vi "Controller Test Bench (4).vi"() -> ()   [LabVIEW 2022 SP3]
uses:
  <vilib>/sound2/lvsound2.llb/Sound Data Format.ctl
  <vilib>/Utility/error.llb/DialogType.ctl
  <vilib>/sound2/lvsound2.llb/Sampling Mode.ctl
  <vilib>/Analysis/4window.llb/windowTd.ctl
  <vilib>/DAQmx/read.llb/DAQmx Read (Analog 1D Wfm NChan NSamp).vi
  <vilib>/DAQmx/write.llb/DAQmx Write (Analog 1D DBL 1Chan NSamp).vi
  <vilib>/DAQmx/create/channels.llb/DAQmx Create Channel (AO-Voltage-Basic).vi
  <vilib>/DAQmx/create/channels.llb/DAQmx Create Channel (AI-Acceleration-Accelerometer).vi
  <vilib>/DAQmx/configure/timing.llb/DAQmx Timing (Sample Clock).vi
  <vilib>/DAQmx/miscellaneous.llb/DAQmx Fill In Error Info.vi
  <vilib>/DAQmx/configure/task.llb/DAQmx Configure Logging (TDMS).vi
  <vilib>/measure/maspectr.llb/FFT Spectrum (Mag-Phase) for N Chan.vi
  <vilib>/sound2/lvsound2.llb/Sound Output Set Volume (Single).vi
  <vilib>/sound2/lvsound2.llb/Sound Output Write (DBL Single).vi
  <vilib>/measure/NI_MAPro.lvlib
  <resource>/objmgr/daqmx.rc
  <vilib>/Analysis/NI_AALPro.lvlib
panel:
  out "number of samples written per channel":u32
  in  "Active Control":bool
  in  "Output Noise":bool
  in  "Log Data":bool
  out "Phase 2":cluster{"f0":dbl, "df":dbl, "phase":dbl[]}[](graph)
  out "Mag 2":cluster{"f0":dbl, "df":dbl, "magnitude":dbl[]}[](graph)
  in  "Show FFT":bool
  in  "Save FFT":bool
  in  "Start Acquisition":bool
  in  "Stop":bool
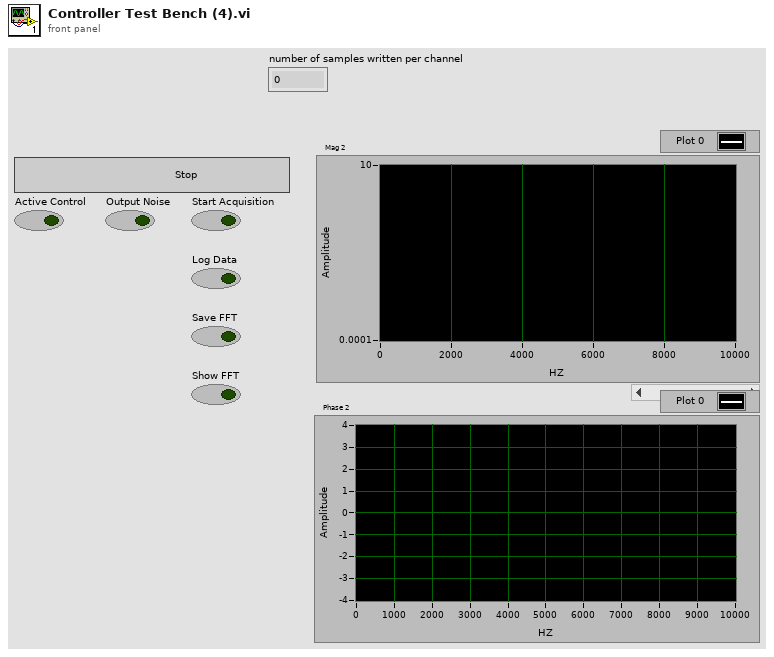
[diagram p1: front panel]
types:
  T1 = typedef "Sampling Mode.ctl" = i32
  T2 = typedef "DialogType.ctl" = u16
  T3 = typedef "Sound Data Format.ctl" = cluster{"sample rate (S/s)":dbl, "number of channels":i32, "bits per sample":i32}
  T4 = typedef "Sound Output Task ID.ctl" = u32
  T5 = typedef "NI_AALPro.lvlib/windowTd.ctl" = u32
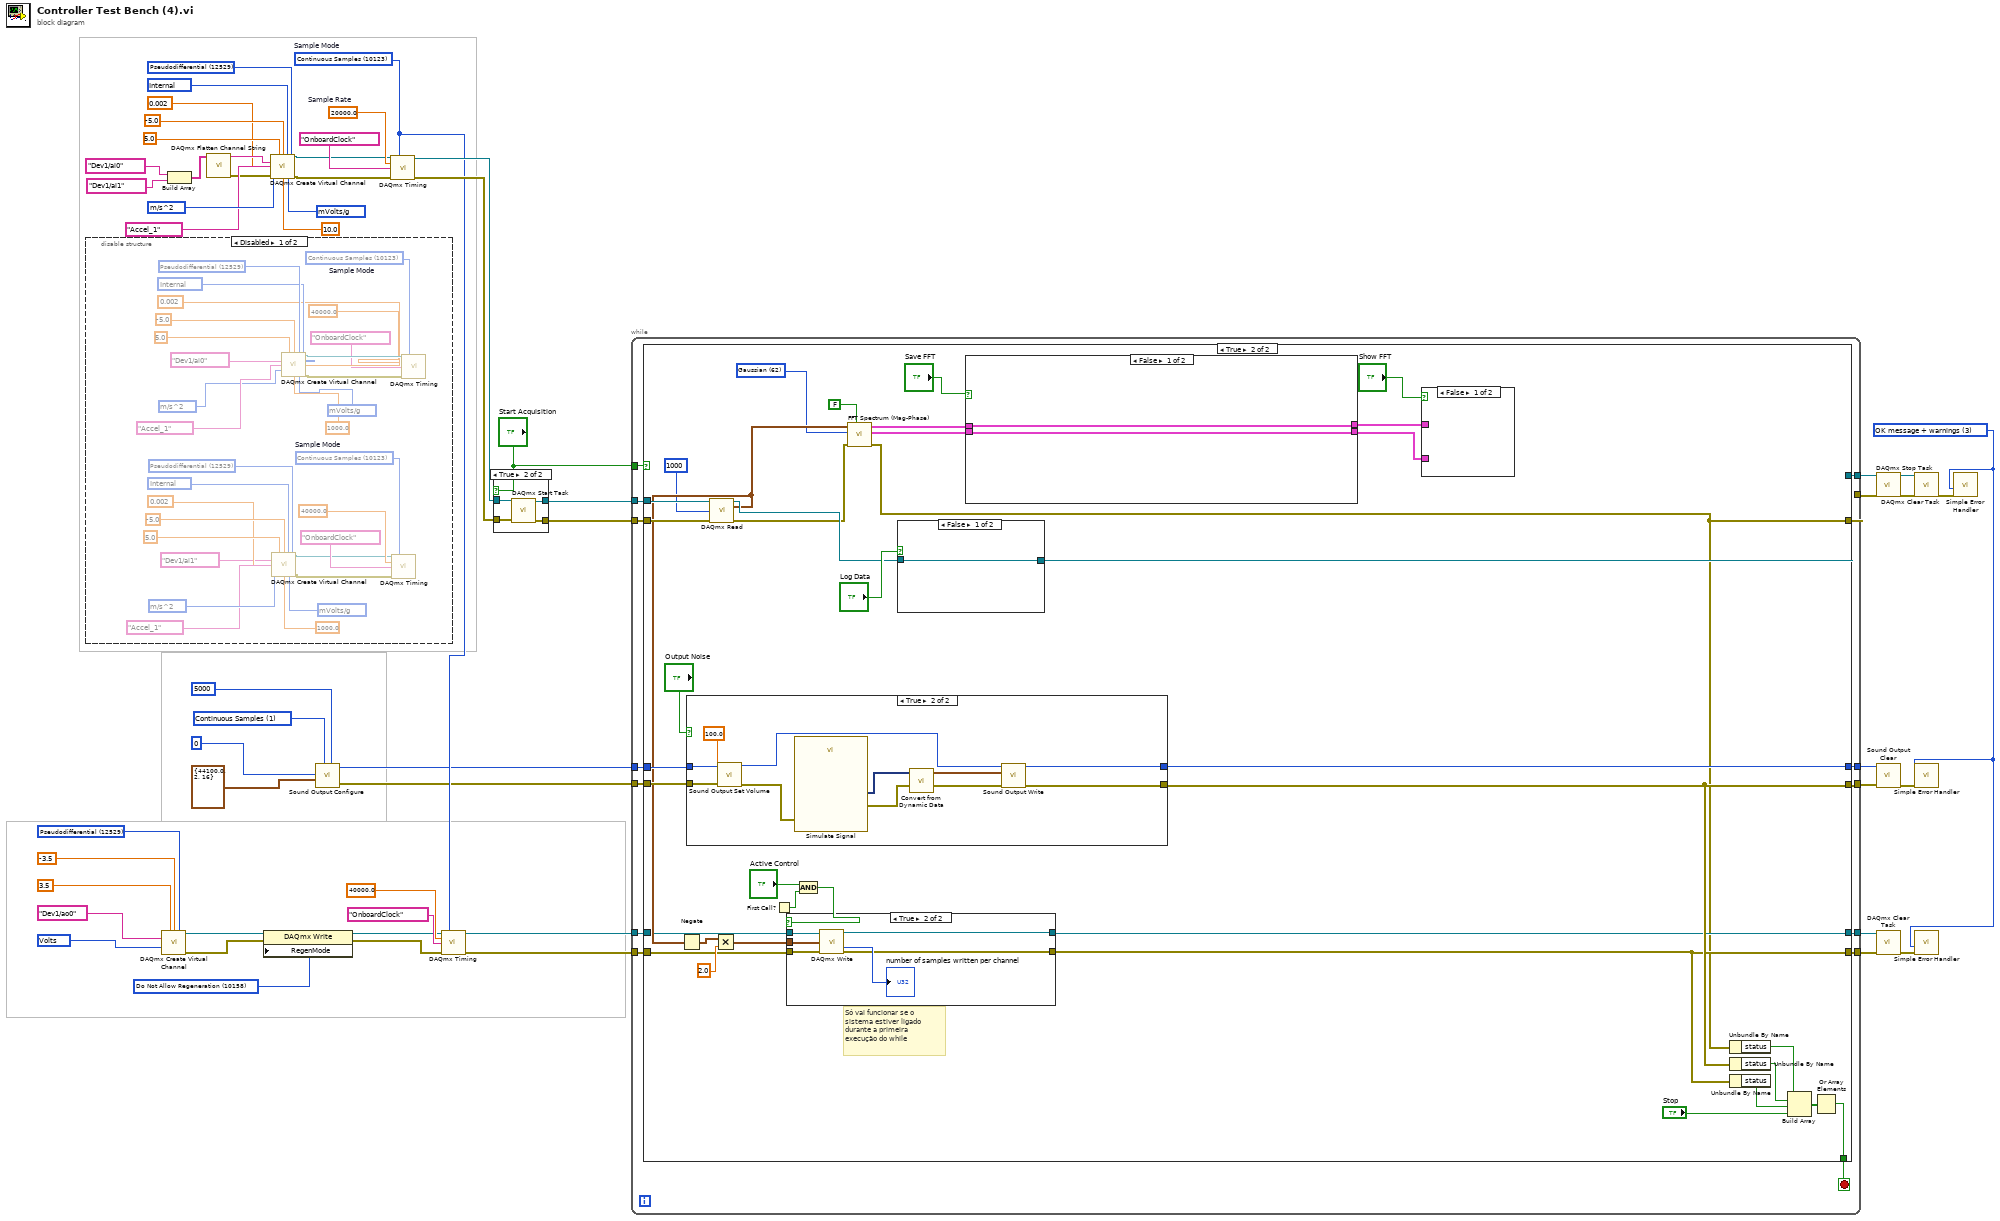
[diagram p0: block diagram]
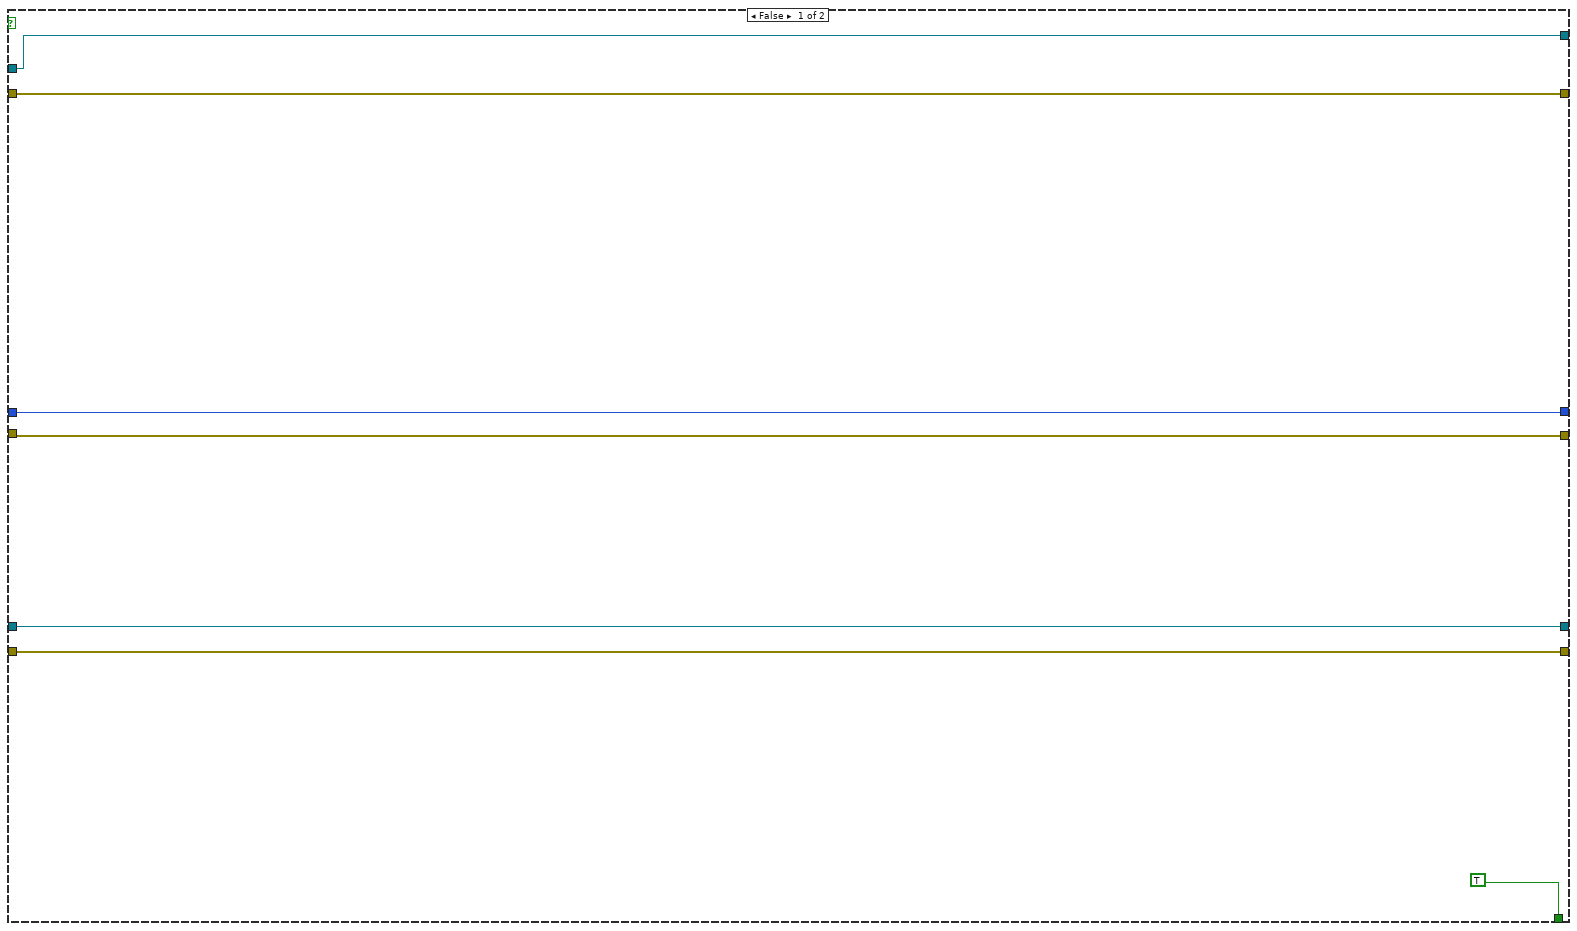
[diagram p4: hidden frame]
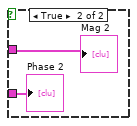
[diagram p7: hidden frame]
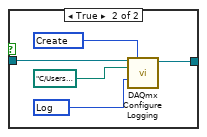
[diagram p9: hidden frame]
diagram:
  w1 = T1 1 items=["Finite Samples", "Continuous Samples"] ("sample mode")
  w15 = 10158 items=["Allow Regeneration"=10097, "Do Not Allow Regeneration"=10158] ("RegenMode")
  w20 = 12509 items=["mVolts/g"=12509, "Volts/g"=12510] ("sensitivity units")
  w23 = 10200 items=["Internal"=10200, "External"=10167, "None"=10230] ("current excitation source")
  w4 = T2 3 items=["no dialog", "OK message", "continue or stop message", "OK message + warnings", "continue/stop + warnings"] ("type of dialog (OK msg:1)")
  w42 = 20000.0  # Sample Rate
  w5 = 10123 items=["Finite Samples"=10178, "Continuous Samples"=10123, "Hardware Timed Single Point"=12522]  # Sample Mode
  w46 = 12529 items=["Default"=-1, "RSE"=10083, "Differential"=10106, "Pseudodifferential"=12529] ("output terminal configuration")
  w44 = 10348 items=["Volts"=10348, "From Custom Scale"=10065] ("units")
  w52 = 12529 items=["default"=-1, "RSE"=10083, "NRSE"=10078, "Differential"=10106, "Pseudodifferential"=12529] ("input terminal configuration")
  w56 = 12470 items=["g"=10186, "m/s^2"=12470, "in/s^2"=12471, "From Custom Scale"=10065] ("units")
  n1 = disable-structure shown="Disabled" {
    frame Disabled {
      w60 = 12509 items=["mVolts/g"=12509, "Volts/g"=12510] ("sensitivity units")
      w65 = 10200 items=["Internal"=10200, "External"=10167, "None"=10230] ("current excitation source")
      w59 = 10123 items=["Finite Samples"=10178, "Continuous Samples"=10123, "Hardware Timed Single Point"=12522]  # Sample Mode
      w67 = 12529 items=["default"=-1, "RSE"=10083, "NRSE"=10078, "Differential"=10106, "Pseudodifferential"=12529] ("input terminal configuration")
      w62 = 12470 items=["g"=10186, "m/s^2"=12470, "in/s^2"=12471, "From Custom Scale"=10065] ("units")
      w73 = 12509 items=["mVolts/g"=12509, "Volts/g"=12510] ("sensitivity units")
      w76 = 10200 items=["Internal"=10200, "External"=10167, "None"=10230] ("current excitation source")
      w81 = 10123 items=["Finite Samples"=10178, "Continuous Samples"=10123, "Hardware Timed Single Point"=12522]  # Sample Mode
      w82 = 12529 items=["default"=-1, "RSE"=10083, "NRSE"=10078, "Differential"=10106, "Pseudodifferential"=12529] ("input terminal configuration")
      w86 = 12470 items=["g"=10186, "m/s^2"=12470, "in/s^2"=12471, "From Custom Scale"=10065] ("units")
      n2 = call-poly <vilib>:"DAQmx Create Virtual Channel.vi"("maximum value"=5.0, "minimum value"=-5.0, "input terminal configuration"=w82, "physical channels"=tag "Dev1/ai1", "current excitation source"=w76, "name to assign"="Accel_1", "current excitation value"=0.002, "units"=w86, "sensitivity"=1000.0, "sensitivity units"=w73) -> ("task out"=w78:refnum<k21>, "error out"=w77:errorcluster)  [unwired: 4 in]
      n3 = call-poly <vilib>:"DAQmx Create Virtual Channel.vi"("maximum value"=5.0, "minimum value"=-5.0, "input terminal configuration"=w67, "physical channels"=tag "Dev1/ai0", "current excitation source"=w65, "name to assign"="Accel_1", "current excitation value"=0.002, "units"=w62, "sensitivity"=1000.0, "sensitivity units"=w60) -> ("task out"=w70:refnum<k21>, "error out"=w71:errorcluster)  [unwired: 4 in]
      n4 = call-poly <vilib>:"DAQmx Timing.vi"("task/channels in"=w78, "sample mode"=w81, "rate"=40000.0 ("Sample Rate"), "source"=tag "OnboardClock" ("Sample Clock Source"), "error in"=w77) -> ()  [unwired: 9 in, 2 out]
      n5 = call-poly <vilib>:"DAQmx Timing.vi"("task/channels in"=w70, "sample mode"=w59, "rate"=40000.0 ("Sample Rate"), "source"=tag "OnboardClock" ("Sample Clock Source"), "error in"=w71) -> ()  [unwired: 9 in, 2 out]
    }
    frame Enabled {
    }
  }
  n6 = call-poly <vilib>:"DAQmx Create Virtual Channel.vi"("maximum value"=3.5, "minimum value"=-3.5, "output terminal configuration"=w46, "physical channels"=tag "Dev1/ao0", "units"=w44) -> ("task out"=w12:refnum<k21>, "error out"=w16:errorcluster)  [unwired: 9 in]
  n7 = Build Array(tag "Dev1/ai0" ("physical channels"), tag "Dev1/ai1" ("physical channels")) -> (w38:tag[])
  n8 = call <vilib>:"DAQmx Flatten Channel String.vi"("names in"=w38) -> ("names out"=w36:string, "error out"=w37:errorcluster)  [unwired: 13 in]
  n9 = property class="DAQmx Write"(reference=w12, error in=w16, "RegenMode"=w15) -> (reference out=w10:refnum<k21>, error out=w11:errorcluster)
  n10 = call-poly <vilib>:"DAQmx Create Virtual Channel.vi"("maximum value"=5.0, "minimum value"=-5.0, "input terminal configuration"=w52, "physical channels"=w36, "current excitation source"=w23, "name to assign"="Accel_1", "current excitation value"=0.002, "units"=w56, "error in"=w37, "sensitivity"=10.0, "sensitivity units"=w20) -> ("task out"=w41:refnum<k21>, "error out"=w40:errorcluster)  [unwired: 3 in]
  n11 = call <vilib>:"Sound Output Configure.vi"("number of samples/ch"=5000 ("Number of Samples/ch"), "sample mode"=w1, "sound format"=T3 {"sample rate (S/s)"=44100.0, "number of channels"=2, "bits per sample"=16} ("Sound Format"), "device ID"=u32 0 ("Device ID")) -> ("error out"=w3:errorcluster, "task ID"=w2:T4)  [unwired: 6 in]
  n12 = call-poly <vilib>:"DAQmx Timing.vi"("task/channels in"=w41, "sample mode"=w5, "rate"=w42, "source"=tag "OnboardClock" ("Sample Clock Source"), "error in"=w40) -> ("task out"=w39:refnum<k21>, "error out"=w19:errorcluster)  [unwired: 9 in]
  n13 = call-poly <vilib>:"DAQmx Timing.vi"("task/channels in"=w10, "sample mode"=w5, "rate"=40000.0 ("Sample Rate"), "source"=tag "OnboardClock" ("Sample Clock Source"), "error in"=w11) -> ("task out"=w14:refnum<k21>, "error out"=w13:errorcluster)  [unwired: 9 in]
  n14 = case shown="True" "Start Acquisition" {
    tunnel: w19 -> [w87 w92]
    tunnel: w39 -> [w88 w91]
    tunnel: [w88 w90] -> w35
    tunnel: [w87 w89] -> w34
    frame False {
    }
    frame True {
      n15 = call <vilib>:"DAQmx Start Task.vi"("task/channels in"=w91, "error in"=w92) -> ("task out"=w90:refnum<k21>, "error out"=w89:errorcluster)  [unwired: 12 in]
    }
  }
  n16 = while {
    tunnel: w3 -> [w106]
    tunnel: w2 -> [w104]
    tunnel: w35 -> [w103]
    tunnel: w34 -> [w102]
    tunnel: [w98] -> w30
    tunnel: [w101] -> w29
    tunnel: [w99] -> w27
    tunnel: [w100] -> w26
    tunnel: w14 -> [w97]
    tunnel: w13 -> [w96]
    tunnel: [w94] -> w9
    tunnel: [w95] -> w8
    tunnel: "Start Acquisition" -> [w93]
    stop <- w105 stop-if-true
    n17 = case shown="True" w93 {
      tunnel: w106 -> [w110 w151]
      tunnel: [TRUE w150] -> w105
      tunnel: w104 -> [w111 w149]
      tunnel: w103 -> [w113 w148]
      tunnel: w102 -> [w112 w147]
      tunnel: [w113 w144] -> w101
      tunnel: [w111 w143] -> w100
      tunnel: [w110 w140] -> w99
      tunnel: [w112 w116] -> w98
      tunnel: w97 -> [w109 w123]
      tunnel: w96 -> [w108 w121]
      tunnel: [w109 w120] -> w95
      tunnel: [w108 w119] -> w94
      frame False {
      }
      frame True {
        w115 = T5 62 items=["Rectangle"=0, "Hanning"=1, "Hamming"=2, "Blackman-Harris"=3, "Exact Blackman"=4, "Blackman"=5, "Flat Top"=6, "4 Term B-Harris "=7, "7 Term B-Harris"=8, "Low Sidelobe"=9, "Blackman Nuttall"=11, "Triangle"=30, "Bartlett-Hanning"=31, "Bohman"=32, "Parzen"=33, "Welch"=34, "Kaiser"=60, "Dolph-Chebyshev"=61, "Gaussian"=62] ("window")
        # "Só vai funcionar se o sistema estiver ligado durante a primeira execução do while"
        n18 = case shown="True" "Output Noise" {
          tunnel: w151 -> [w166 w171]
          tunnel: w149 -> [w167 w172]
          tunnel: [w167 w174] -> w143
          tunnel: [w166 w173] -> w140
          frame False {
          }
          frame True {
            n19 = call-poly <vilib>:"Sound Output Set Volume.vi"("error in (no error)"=w171, "volume"=100.0, "task ID"=w172) -> ("error out"=w170:errorcluster, "task ID out"=w169:T4)  [unwired: 7 in]
            n20 = call "Simulate Signal"("error in (no error)"=w170) -> ("DC with Gaussian Noise"=w177:dynamicdata, "error out"=w176:errorcluster)  [unwired: 13 in]
            n21 = call "Convert from Dynamic Data"("Dynamic Data Type"=w177) -> ("Waveform"=w175:waveform(dbl))  [unwired: 3 in]
            n22 = call-poly <vilib>:"Sound Output Write.vi"("error in (no error)"=w176, "data"=w175, "task ID"=w169) -> ("error out"=w173:errorcluster, "task ID out"=w174:T4)  [unwired: 7 in]
          }
        }
        n23 = call-poly <vilib>:"DAQmx Read.vi"("task/channels in"=w148, "number of samples per channel"=1000, "error in"=w147) -> ("task out"=w145:refnum<k21>, "data"=w129:waveform(dbl)[], "error out"=w117:errorcluster)  [unwired: 10 in]
        n24 = Negate(x=w129) -> (-x=w130:waveform(dbl)[])
        n25 = Multiply(x=w130, y=2.0) -> (x*y=w122:waveform(dbl)[])
        n26 = First Call?() -> (First Call?: T/F=w132:bool)
        n27 = And(x="Active Control", y=w132) -> (x .and. y?=w127:bool)
        n28 = case shown="True" w127 {
          tunnel: w121 -> [w153 w157]
          tunnel: [w152 w154] -> w120
          tunnel: [w153 w155] -> w119
          tunnel: w123 -> [w152 w159]
          tunnel: w122 -> [_ w158]
          frame False {
          }
          frame True {
            n29 = call-poly <vilib>:"DAQmx Write.vi"("task/channels in"=w159, "data"=w158, "error in"=w157) -> ("task out"=w154:refnum<k21>, "number of samples written per channel"=→"number of samples written per channel":u32, "error out"=w155:errorcluster)  [unwired: 10 in]
          }
        }
        n30 = call-poly <vilib>:"FFT Spectrum (Mag-Phase).vi"("restart averaging (F)"=FALSE, "error in (no error)"=w117, "window"=w115, "time signals"=w129) -> ("error out"=w116:errorcluster, "phases"=w135:cluster{"f0":dbl, "df":dbl, "phase":dbl[]}[], "magnitudes"=w136:cluster{"f0":dbl, "df":dbl, "magnitude":dbl[]}[])  [unwired: 3 in, 2 out]
        n31 = case shown="False" "Log Data" {
          tunnel: w145 -> [w178 w180]
          tunnel: [w178 w179] -> w144
          frame False {
          }
          frame True {
            w181 = 15848 items=["Open"=10437, "Open or Create"=15846, "Create or Replace"=15847, "Create"=15848] ("operation")
            w182 = 15844 items=["Off"=10231, "Log"=15844, "Log and Read"=15842] ("logging mode")
            n32 = call-poly <vilib>:"DAQmx Configure Logging.vi"("task/channels in"=w180, "operation"=w181, "file path"=path "C:/Users/LAV-UFSC/Documents/LAV - TCC", "logging mode"=w182) -> ("task out"=w179:refnum<k21>)  [unwired: 10 in, 1 out]
          }
        }
        n33 = case shown="False" "Save FFT" {
          tunnel: w136 -> [w160 w163]
          tunnel: w135 -> [w161 w162]
          tunnel: [w161 w162] -> w134
          tunnel: [w160 w163] -> w131
          frame False {
          }
          frame True {
          }
        }
        n34 = case shown="False" "Show FFT" {
          tunnel: w131 -> [_ w165]
          tunnel: w134 -> [_ w164]
          frame False {
          }
          frame True {
            "Mag 2" <- w165
            "Phase 2" <- w164
          }
        }
        n35 = Unbundle By Name(w116) -> ("status"=w126:bool)
        n36 = Unbundle By Name(w140) -> ("status"=w125:bool)
        n37 = Unbundle By Name(w119) -> ("status"=w124:bool)
        n38 = Build Array(w126, w125, w124, "Stop") -> (w141:bool[])
        n39 = Or Array Elements(Boolean array=w141) -> (logical OR=w150:bool)
      }
    }
  }
  n40 = call <vilib>:"DAQmx Stop Task.vi"("task/channels in"=w29, "error in"=w30) -> ("task out"=w32:refnum<k21>, "error out"=w31:errorcluster)  [unwired: 12 in]
  n41 = call <vilib>:"Sound Output Clear.vi"("error in (no error)"=w27, "task ID"=w26) -> ("error out"=w25:errorcluster)  [unwired: 9 in]
  n42 = call <vilib>:"DAQmx Clear Task.vi"("task in"=w8, "error in"=w9) -> ("error out"=w7:errorcluster)  [unwired: 13 in]
  n43 = call <vilib>:"DAQmx Clear Task.vi"("task in"=w32, "error in"=w31) -> ("error out"=w33:errorcluster)  [unwired: 13 in]
  n44 = call <vilib>:"Simple Error Handler.vi"("type of dialog (OK msg:1)"=w4, "error in (no error)"=w25) -> ()  [unwired: 3 in, 5 out]
  n45 = call <vilib>:"Simple Error Handler.vi"("type of dialog (OK msg:1)"=w4, "error in (no error)"=w7) -> ()  [unwired: 3 in, 5 out]
  n46 = call <vilib>:"Simple Error Handler.vi"("type of dialog (OK msg:1)"=w4, "error in (no error)"=w33) -> ()  [unwired: 3 in, 5 out]
